vi "Get Test information.vi"(8 "error in (no error)":errorcluster caption="错误输入（无错误）", 11 "appended path":path) -> (0 "error out":errorcluster caption="错误输出", 2 "数组":string[](array[string]), 3 "appended path 2":path)   [LabVIEW 2018]
uses:
  <vilib>/Utility/config.llb/Read Key (String).vi
  <vilib>/Utility/config.llb/NI_LVConfig.lvlib
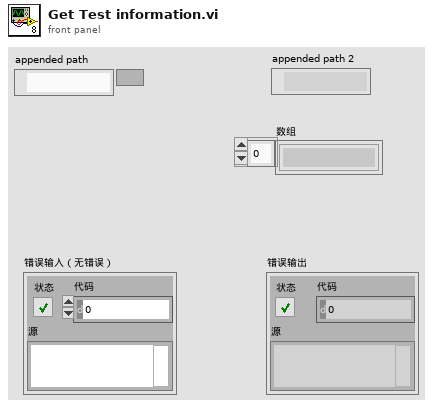
[diagram p1: front panel]
types:
  T1 = typedef "NI_LVConfig.lvlib/Config Data RefNum.ctl" = refnum<k1>
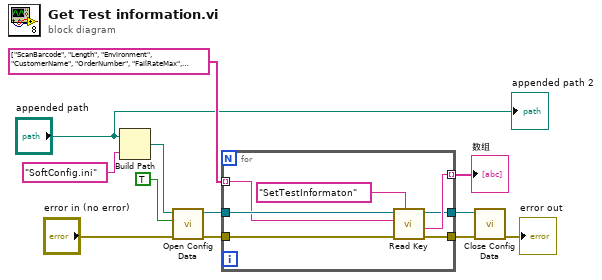
[diagram p0: block diagram]
diagram:
  n1 = Build Path(base path="appended path", name or relative path="SoftConfig.ini" ("名称或相对路径")) -> (appended path=w7:path)
  n2 = call <vilib>:"Open Config Data.vi"("error in (no error)"="error in (no error)", "create file if necessary (T)"=TRUE, "configuration file path"=w7) -> ("error out"=w2:errorcluster, "refnum"=w10:T1)  [unwired: 6 in, 1 out]
  n3 = for {
    tunnel: w10 -> [w19]
    tunnel: [w17] -> w8 mode=indexing
    tunnel: [w16] -> w12
    tunnel: string[] ["ScanBarcode", "Length", "Environment", "CustomerName", "OrderNumber", "FailRateMax", "Inspector", "Repeat"] -> [w15] mode=indexing
    tunnel: [w14] -> w3
    tunnel: w2 -> [w13]
    n4 = call-poly <vilib>:"Read Key.vi"("section"="SetTestInformaton", "error in (no error)"=w13, "key"=w15, "refnum"=w19) -> ("error out"=w14:errorcluster, "value"=w17:string, "refnum out"=w16:T1)  [unwired: 4 in, 1 out]
  }
  "数组" <- w8
  n5 = call <vilib>:"Close Config Data.vi"("error in (no error)"=w3, "refnum"=w12) -> ("error out"=→"error out":errorcluster)  [unwired: 8 in, 1 out]
  "appended path 2" <- "appended path"
